vi "Untitled tttttt.vi"() -> ()   [LabVIEW 2010]
uses:
  Defenitions/LEIN Structure variations.ctl
  Defenitions/LEIN CMD List.ctl
  Defenitions/LEIN CMD Cluster.ctl
panel:
  in  "array 2":u8[](array[numeric])
  out "STAT Part 2":u8
  out "STAT ID 2":u8
  out "Data":u8[](array[numeric])
  out "SID 2":u8
  in  "STAT Part":u8
  in  "STAT ID":u8
  in  "SID":u8
  out "LEIN OK 2":bool
  out "LEIN OK":bool
  in  "array":u8[](array[numeric])
  out "error out 2":errorcluster
  out "error out":errorcluster
  out "CMD out 2":T1={"SID"=0, "ANF"=FALSE, "CMD"=enum."TASK", "DATA"=[]}
  out "CMD out":T1={"SID"=0, "ANF"=FALSE, "CMD"=enum."TASK", "DATA"=[]}
  out "LEIN Frame":bool
  out "CMD 2":T1={"SID"=0, "ANF"=FALSE, "CMD"=enum."TASK", "DATA"=[]}
  in  "CMD":T1={"SID"=0, "ANF"=FALSE, "CMD"=enum."TASK", "DATA"=[]}
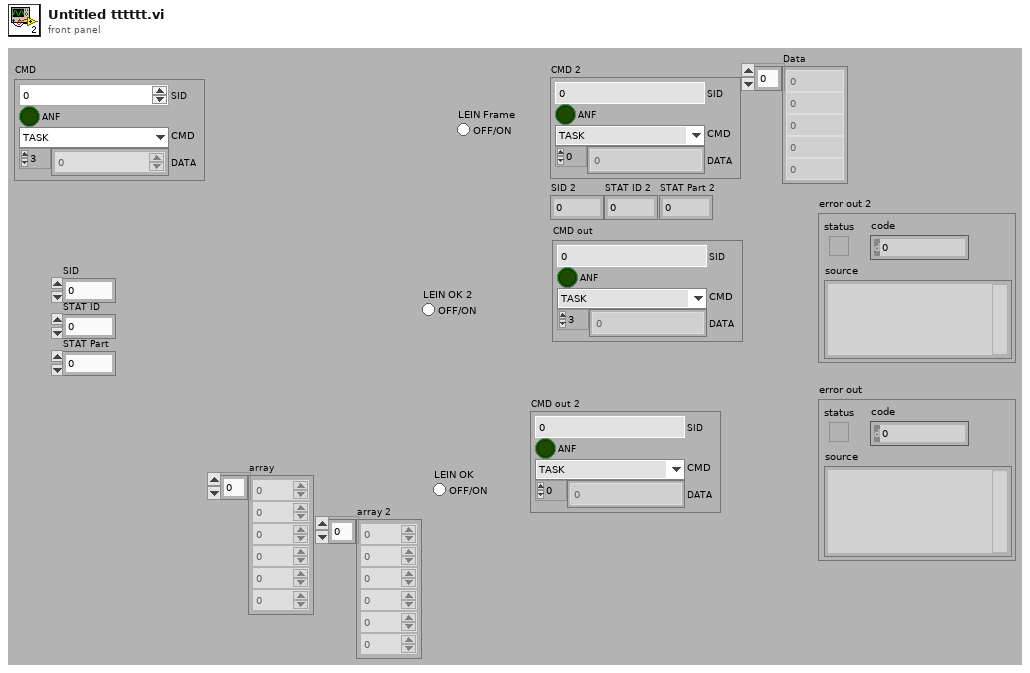
[diagram p1: front panel]
types:
  T1 = typedef "LEIN CMD Cluster.ctl" = cluster{"SID":u8, "ANF":bool, "CMD":T2, "DATA":u8[]}
  T2 = typedef "LEIN CMD List.ctl" = enum8{"ACTI", "TASK", "RES0", "STAT", "RES1", "RES2", "RES3", "USER"}
  T3 = typedef "LEIN Structure variations.ctl" = enum16{"LEIN08", "LEIN31", "LEIN63"}
  T4 = typedef "CanFrameTimed.ctl" = cluster{"Timestamp":dbl, "ArbitrationId":u32, "IsRemote":u8, "DataLength":u8, "Data":u8[]}
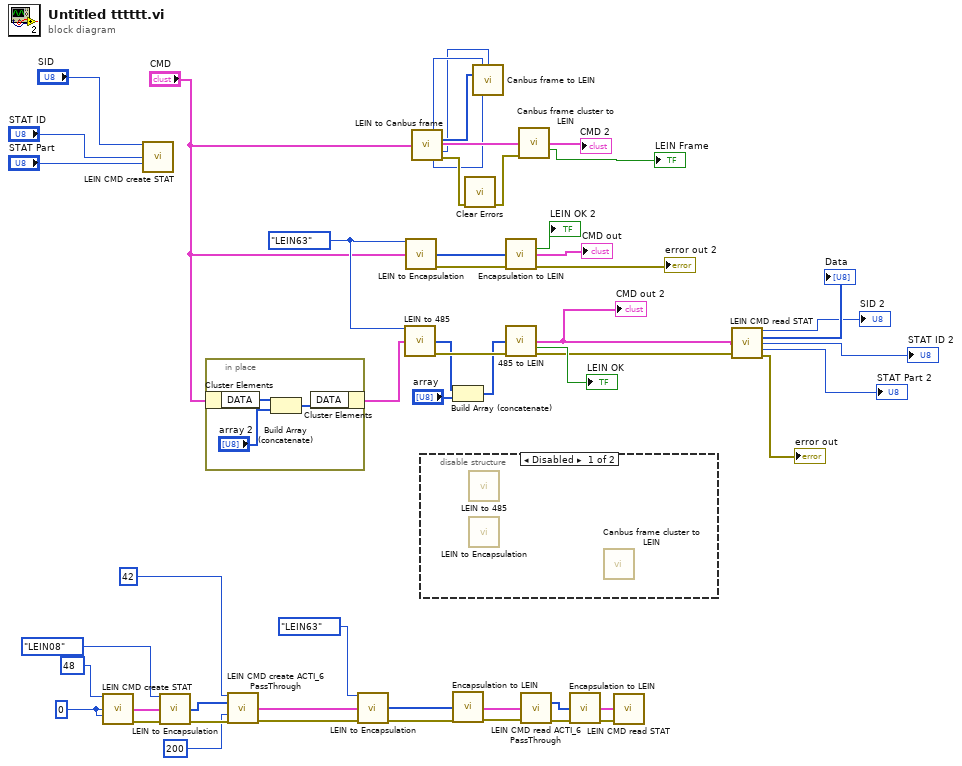
[diagram p0: block diagram]
diagram:
  w19 = u8 0 ("STAT ID")
  w43 = LEIN_Structure_variations."LEIN63" ("LEIN Variation")
  n1 = call "LEIN CMD create STAT.vi"("SID"=u8 48, "STAT ID"=w19, "STAT Part"=w19) -> ("CMD"=w17:T1, "error out"=w18:errorcluster)  [unwired: 11 in]
  n2 = call "LEIN CMD create STAT.vi"("SID"="SID", "STAT ID"="STAT ID", "STAT Part"="STAT Part") -> ()  [unwired: 11 in, 2 out]
  n3 = call "LEIN to Encapsulation.vi"("LEIN Variation"=LEIN_Structure_variations."LEIN08", "CMD"=w17, "error in (no error)"=w18) -> ("Data and header"=w14:u8[], "error out"=w15:errorcluster)  [unwired: 8 in, 3 out]
  n4 = in-place {
    n5 = in-place-cluster #1("CMD") -> ("DATA"=w54:u8[])
    n6 = Build Array (concatenate)(w54, "array 2") -> (w53:u8[])
    n7 = in-place-cluster #1("DATA"=w53) -> (w21:T1)
  }
  n8 = call "LEIN CMD create ACTI_6 PassThrough.vi"("SID"=u8 42, "LEIN ecapsulated data (header and data)"=w14, "Sub Timeout (ms)"=u16 200, "error in (no error)"=w15) -> ("CMD"=w9:T1, "error out"=w11:errorcluster)  [unwired: 10 in]
  n9 = call "LEIN to Encapsulation.vi"("LEIN Variation"=LEIN_Structure_variations."LEIN63", "CMD"=w9, "error in (no error)"=w11) -> ("Data and header"=w7:u8[], "error out"=w8:errorcluster)  [unwired: 8 in, 3 out]
  n10 = call "LEIN to 485.vi"("LEIN Variation"=w43, "CMD"=w21) -> ("Data  header and CRC"=w38:u8[], "error out"=w42:errorcluster)  [unwired: 7 in, 5 out]
  n11 = call "LEIN to Encapsulation.vi"("LEIN Variation"=w43, "CMD"="CMD") -> ("Data and header"=w40:u8[], "error out"=w41:errorcluster)  [unwired: 9 in, 3 out]
  n12 = call "LEIN to Canbus frame.vi"("CMD"="CMD") -> ("Data Length"=w45:u32, "Data"=w46:u8[], "Complete frame"=w48:T4, "Is remote"=w44:u8, "ArbitrationID"=w47:u32, "error out"=w52:errorcluster)  [unwired: 9 in]
  n13 = disable-structure shown="Disabled" {
    frame Disabled {
      n14 = call "LEIN to 485.vi"() -> ()  [unwired: 9 in, 7 out]
      n15 = call "LEIN to Encapsulation.vi"() -> ()  [unwired: 11 in, 5 out]
      n16 = call "Canbus frame cluster to LEIN.vi"() -> ()  [unwired: 13 in, 3 out]
    }
    frame Enabled {
    }
  }
  n17 = Build Array (concatenate)(w38, "array") -> (w37:u8[])
  n18 = call "Encapsulation to LEIN.vi"("Data and header"=w7, "error in (no error)"=w8) -> ("CMD out"=w5:T1, "error out"=w6:errorcluster)  [unwired: 10 in, 2 out]
  n19 = call <vilib>:"Clear Errors.vi"("error in (no error)"=w52) -> ("error out"=w51:errorcluster)  [unwired: 6 in]
  n20 = call "Canbus frame to LEIN.vi"("Data Length"=w45, "IsRemote(0)"=w44, "Data"=w46, "ArbitrationID"=w47) -> ()  [unwired: 9 in, 3 out]
  n21 = call "Encapsulation to LEIN.vi"("Data and header"=w40, "error in (no error)"=w41) -> ("LEIN OK"=→"LEIN OK 2":bool, "CMD out"=→"CMD out":T1, "error out"=→"error out 2":errorcluster)  [unwired: 10 in, 1 out]
  n22 = call "485 to LEIN.vi"("Header, data, CRC"=w37, "error in (no error)"=w42) -> ("CMD out"=w23:T1, "LEIN OK"=→"LEIN OK":bool, "error out"=w25:errorcluster)  [unwired: 11 in]
  "CMD out 2" <- w23
  n23 = call "Canbus frame cluster to LEIN.vi"("CAN FRAME TIMED"=w48, "error in (no error)"=w51) -> ("CMD"=→"CMD 2":T1, "LEIN Frame"=→"LEIN Frame":bool)  [unwired: 11 in, 1 out]
  n24 = call "LEIN CMD read ACTI_6 PassThrough.vi"("CMD"=w5, "error in (no error)"=w6) -> ("Reply from sub ID"=w3:u8[], "error out"=w4:errorcluster)  [unwired: 10 in, 2 out]
  n25 = call "Encapsulation to LEIN.vi"("Data and header"=w3, "error in (no error)"=w4) -> ("CMD out"=w1:T1, "error out"=w2:errorcluster)  [unwired: 10 in, 2 out]
  n26 = call "LEIN CMD read STAT.vi"("CMD"=w1, "error in (no error)"=w2) -> ()  [unwired: 8 in, 6 out]
  n27 = call "LEIN CMD read STAT.vi"("CMD"=w23, "error in (no error)"=w25) -> ("SID"=→"SID 2":u8, "Data"=→"Data":u8[], "STAT ID"=→"STAT ID 2":u8, "STAT Part"=→"STAT Part 2":u8, "error out"=→"error out":errorcluster)  [unwired: 8 in, 1 out]
